vi "DCPower Model to Ranges.vi"(0 "SMU Model":string, 5 "Channel":string="0") -> (4 "Voltage Ranges (V)":dbl[](array[numeric]) format="%#_6p", 6 "Current Ranges (A)":dbl[](array[numeric]) format="%#_6p", 8 "Output Resistance Ranges (Ohms)":dbl[](array[numeric]) format="%#_6p")   [LabVIEW 2020]
doc: "This VI takes a DCPower Model Number (such as \"4139\") and outputs it's Voltage, Current, and Output Resistance (if supported) ranges.\n\nFor devices that don't support Output Resistance, the array returned will be empty for the ranges."
panel:
  # "4 Numeric Digits of the model\n\ne.g. \"4139\""
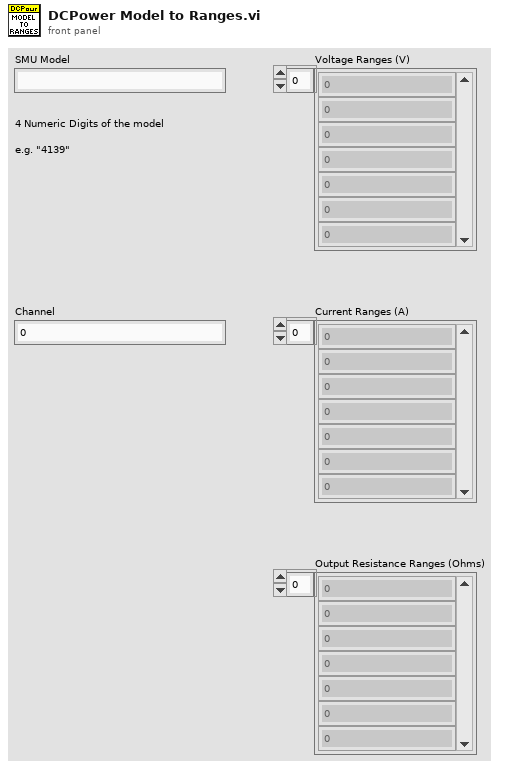
[diagram p1: front panel]
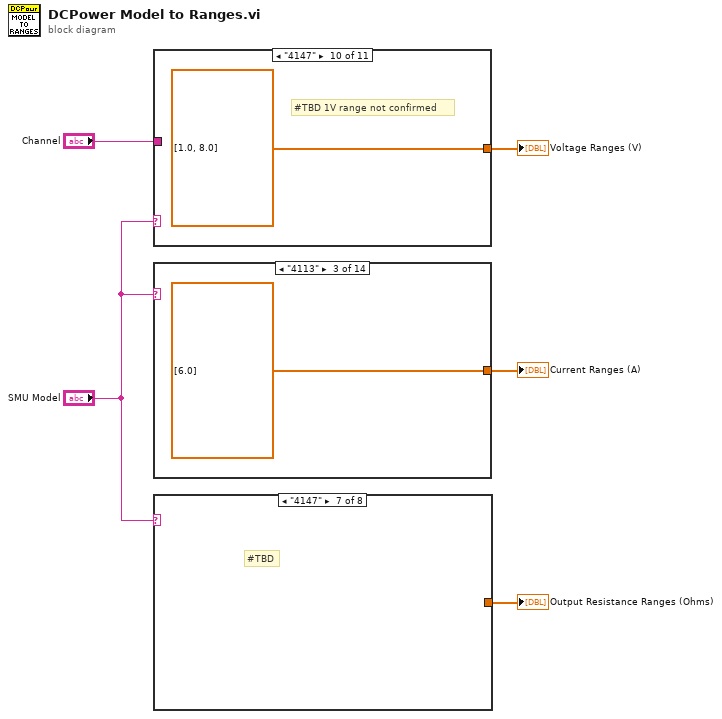
[diagram p0: block diagram]
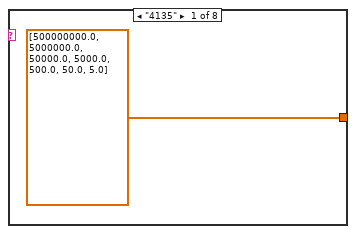
[diagram p2: hidden frame]
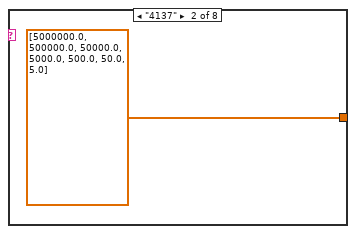
[diagram p3: hidden frame]
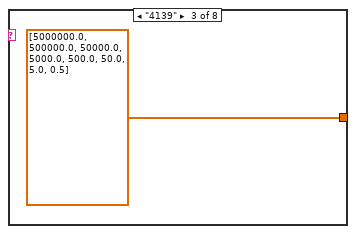
[diagram p4: hidden frame]
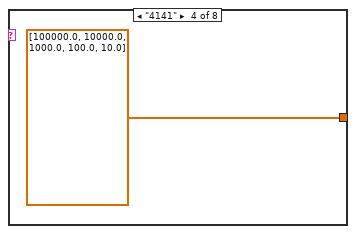
[diagram p5: hidden frame]
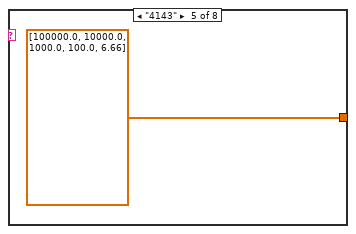
[diagram p6: hidden frame]
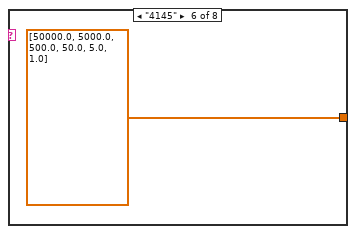
[diagram p7: hidden frame]
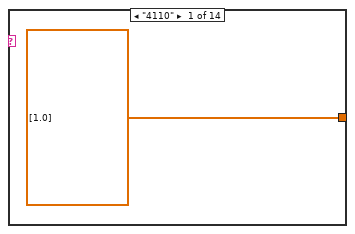
[diagram p9: hidden frame]
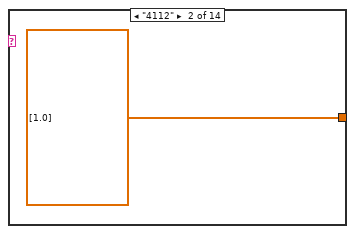
[diagram p10: hidden frame]
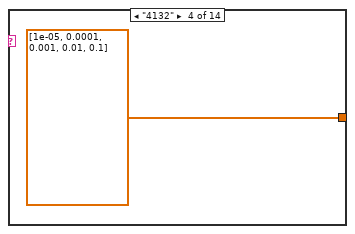
[diagram p11: hidden frame]
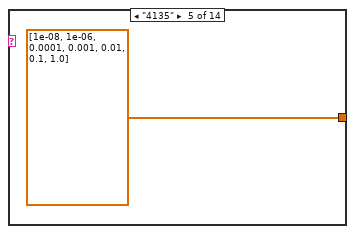
[diagram p12: hidden frame]
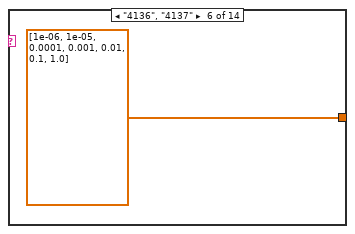
[diagram p13: hidden frame]
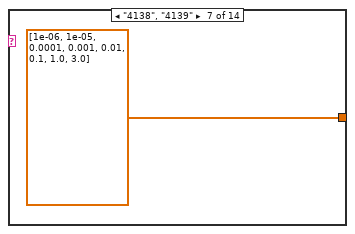
[diagram p14: hidden frame]
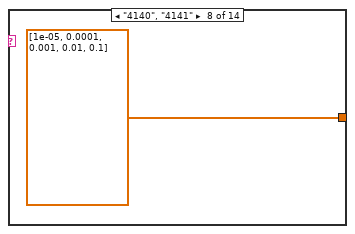
[diagram p15: hidden frame]
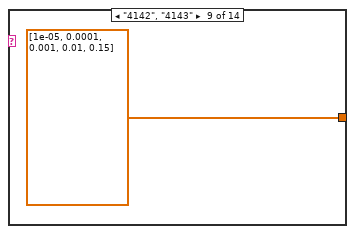
[diagram p16: hidden frame]
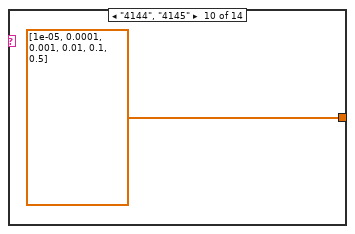
[diagram p17: hidden frame]
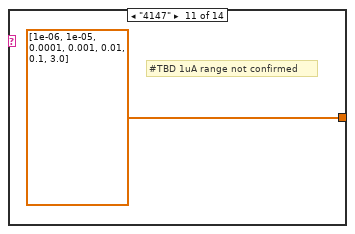
[diagram p18: hidden frame]
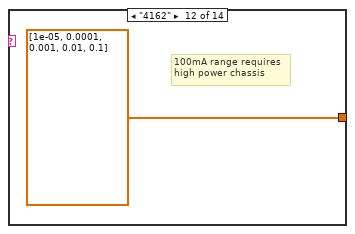
[diagram p19: hidden frame]
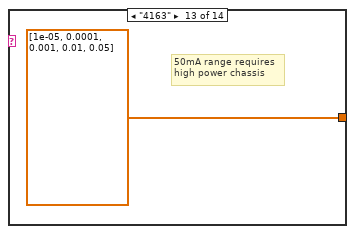
[diagram p20: hidden frame]
diagram:
  n1 = case shown="\"4147\"" "SMU Model" {
    tunnel: [w6 dbl[] [60.0] dbl[] [10.0] dbl[] [10.0, 100.0] dbl[] [0.6, 6.0, 20.0, 200.0] dbl[] [0.6, 6.0, 60.0] dbl[] [10.0] dbl[] [24.0] dbl[] [6.0] dbl[] [1.0, 8.0] _] -> w5
    tunnel: "Channel" -> [w7 _ _ _ _ _ _ _ _ _ _]
    frame "4110" {
      n2 = case shown="\"2\"" w7 {
        tunnel: [_ w8 w10 w12] -> w6
        frame Default {
        }
        frame "0" {
          n3 = Build Array(6.0) -> (w8:dbl[])
        }
        frame "1" {
          n4 = Build Array(20.0) -> (w10:dbl[])
        }
        frame "2" {
          n5 = Build Array(-20.0) -> (w12:dbl[])
        }
      }
    }
    frame "4112" {
    }
    frame "4113" {
    }
    frame "4132" {
    }
    frame "4135", "4136", "4137" {
    }
    frame "4138", "4139" {
    }
    frame "4140", "4141" {
    }
    frame "4142", "4143", "4162", "4163" {
    }
    frame "4144", "4145" {
    }
    frame "4147" {
      # "#TBD 1V range not confirmed"
    }
    frame Default {
    }
  }
  "Voltage Ranges (V)" <- w5
  n6 = case shown="\"4113\"" "SMU Model" {
    tunnel: [dbl[] [1.0] dbl[] [1.0] dbl[] [6.0] dbl[] [1e-05, 0.0001, 0.001, 0.01, 0.1] dbl[] [1e-08, 1e-06, 0.0001, 0.001, 0.01, 0.1, 1.0] dbl[] [1e-06, 1e-05, 0.0001, 0.001, 0.01, 0.1, 1.0] dbl[] [1e-06, 1e-05, 0.0001, 0.001, 0.01, 0.1, 1.0, 3.0] dbl[] [1e-05, 0.0001, 0.001, 0.01, 0.1] dbl[] [1e-05, 0.0001, 0.001, 0.01, 0.15] dbl[] [1e-05, 0.0001, 0.001, 0.01, 0.1, 0.5] dbl[] [1e-06, 1e-05, 0.0001, 0.001, 0.01, 0.1, 3.0] dbl[] [1e-05, 0.0001, 0.001, 0.01, 0.1] dbl[] [1e-05, 0.0001, 0.001, 0.01, 0.05] _] -> w4
    frame "4110" {
    }
    frame "4112" {
    }
    frame "4113" {
    }
    frame "4132" {
    }
    frame "4135" {
    }
    frame "4136", "4137" {
    }
    frame "4138", "4139" {
    }
    frame "4140", "4141" {
    }
    frame "4142", "4143" {
    }
    frame "4144", "4145" {
    }
    frame "4147" {
      # "#TBD 1uA range not confirmed"
    }
    frame "4162" {
      # "100mA range requires\nhigh power chassis"
    }
    frame "4163" {
      # "50mA range requires\nhigh power chassis"
    }
    frame Default {
    }
  }
  "Current Ranges (A)" <- w4
  n7 = case shown="\"4147\"" "SMU Model" {
    tunnel: [dbl[] [500000000.0, 5000000.0, 50000.0, 5000.0, 500.0, 50.0, 5.0] dbl[] [5000000.0, 500000.0, 50000.0, 5000.0, 500.0, 50.0, 5.0] dbl[] [5000000.0, 500000.0, 50000.0, 5000.0, 500.0, 50.0, 5.0, 0.5] dbl[] [100000.0, 10000.0, 1000.0, 100.0, 10.0] dbl[] [100000.0, 10000.0, 1000.0, 100.0, 6.66] dbl[] [50000.0, 5000.0, 500.0, 50.0, 5.0, 1.0] _ _] -> w2
    frame "4135" {
    }
    frame "4137" {
    }
    frame "4139" {
    }
    frame "4141" {
    }
    frame "4143" {
    }
    frame "4145" {
    }
    frame "4147" {
      # "#TBD"
    }
    frame Default {
    }
  }
  "Output Resistance Ranges (Ohms)" <- w2
